vi "JSRKeyboardControl.vi"(8 "PlatMods":T1, 10 "Char":i16, 11 "JSR Simple":refnum<vi>) -> ()   [LabVIEW 2022 SP3]
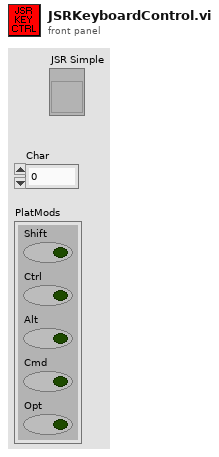
[diagram p1: front panel]
types:
  T1 = cluster{"Shift":bool, "Ctrl":bool, "Alt":bool, "Cmd":bool, "Opt":bool}
  T2 = typedef "JSR Simple.ctl" = cluster{"Pulse Energy Level":T3, "Gain (dB)":T4, "Pulser Voltage (V)":T5}
  T3 = typedef "Energy.ctl" = u16
  T4 = typedef "Gain.ctl" = i8
  T5 = typedef "Volt.ctl" = i16
  T6 = typedef "LVStringsAndValuesArrayTypeDef_U16.ctl" = cluster{"String":string, "Value":u16}[]
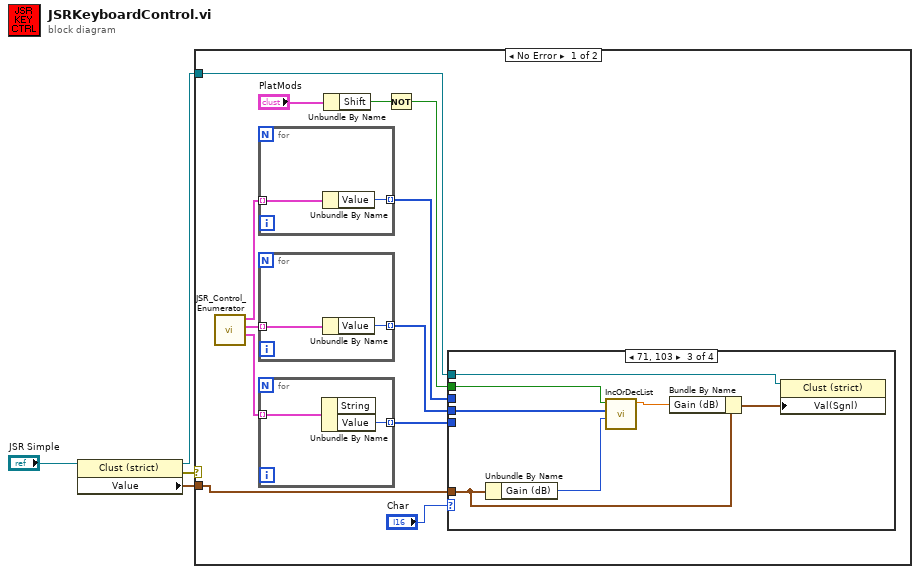
[diagram p0: block diagram]
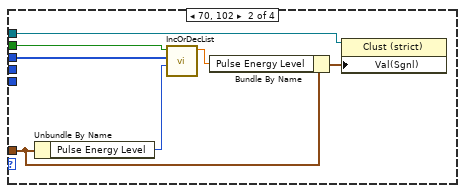
[diagram p3: hidden frame]
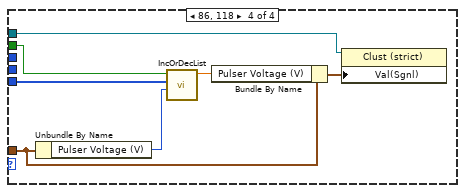
[diagram p4: hidden frame]
diagram:
  n1 = property on="Property Node" class="Clust (strict)"(reference="JSR Simple") -> (reference out=w3:refnum<vi>, error out=w2:errorcluster, "Value"=w4:T2)  [unwired: 1 in]
  n2 = case shown="No Error" w2 {
    tunnel: w4 -> [w14 _]
    tunnel: w3 -> [w13 _]
    frame No Error {
      n3 = call "JSR_Control_Enumerator.vi"() -> ("Voltage"=w10:T6, "Gain"=w9:T6, "Pulse Energy Level"=w8:T6)  [unwired: 9 in]
      n4 = for {
        tunnel: w8 -> [w18] mode=indexing
        tunnel: [w17] -> w6 mode=indexing
        n5 = Unbundle By Name(w18) -> ("Value"=w17:u16)
      }
      n6 = for {
        tunnel: w9 -> [w20] mode=indexing
        tunnel: [w19] -> w7 mode=indexing
        n7 = Unbundle By Name(w20) -> ("Value"=w19:u16)
      }
      n8 = for {
        tunnel: w10 -> [w43] mode=indexing
        tunnel: [w42] -> w11 mode=indexing
        n9 = Unbundle By Name(w43) -> ("Value"=w42:u16)  [unwired: 1 out]
      }
      n10 = Unbundle By Name("PlatMods") -> ("Shift"=w12:bool)
      n11 = Not(x=w12) -> (.not. x?=w5:bool)
      n12 = case shown="71, 103" "Char" {
        tunnel: w14 -> [_ w27 w34 w41]
        tunnel: w13 -> [_ w25 w32 w39]
        tunnel: w5 -> [_ w21 w30 w37]
        tunnel: w11 -> [_ _ _ w36]
        tunnel: w7 -> [_ _ w29 _]
        tunnel: w6 -> [_ w22 _ _]
        frame Default {
        }
        frame 70, 102 {
          n13 = Unbundle By Name(w27) -> ("Pulse Energy Level"=w24:T3)
          n14 = call "IncOrDecList.vi"("Input"=w24, "Vals"=w22, "Shift"=w21) -> ("Output"=w23:dbl)  [unwired: 8 in]
          n15 = Bundle By Name(cluster=w27, "Pulse Energy Level"=w23) -> (w26:T2)
          n16 = property class="Clust (strict)"(reference=w25, "Val(Sgnl)"=w26) -> ()  [unwired: 1 in, 2 out]
        }
        frame 71, 103 {
          n17 = Unbundle By Name(w34) -> ("Gain (dB)"=w28:T4)
          n18 = call "IncOrDecList.vi"("Input"=w28, "Vals"=w29, "Shift"=w30) -> ("Output"=w31:dbl)  [unwired: 8 in]
          n19 = Bundle By Name(cluster=w34, "Gain (dB)"=w31) -> (w33:T2)
          n20 = property class="Clust (strict)"(reference=w32, "Val(Sgnl)"=w33) -> ()  [unwired: 1 in, 2 out]
        }
        frame 86, 118 {
          n21 = Unbundle By Name(w41) -> ("Pulser Voltage (V)"=w35:T5)
          n22 = call "IncOrDecList.vi"("Input"=w35, "Vals"=w36, "Shift"=w37) -> ("Output"=w38:dbl)  [unwired: 8 in]
          n23 = Bundle By Name(cluster=w41, "Pulser Voltage (V)"=w38) -> (w40:T2)
          n24 = property class="Clust (strict)"(reference=w39, "Val(Sgnl)"=w40) -> ()  [unwired: 1 in, 2 out]
        }
      }
    }
    frame Error {
    }
  }
